vi "Analog Trigger with Interleaving Select.vi"(0 "all channels":cluster{fxp<+/-,12,1>[]}[](array[cluster])=[{[0.0, 0.0, 0.0, 0.0, 0.0, 0.0, 0.0, 0.0, 0.0, 0.0, 0.0, 0.0, 0.0, 0.0, 0.0, 0.0]}, {[0.0, 0.0, 0.0, 0.0, 0.0, 0.0, 0.0, 0.0, 0.0, 0.0, 0.0, 0.0, 0.0, 0.0, 0.0, 0.0]}], 1 "interleaving factor":u16, 5 "channel":fxp<+,2,2> format="%#_4g", 7 "trigger level":fxp<+/-,32,1>, 9 "hysteresis level":fxp<+/-,32,1>, 11 "rising edge":bool=TRUE) -> (4 "all channels delayed":cluster{fxp<+/-,12,1>[]}[](array[cluster]), 6 "triggered":bool)   [LabVIEW 2020, in "GettingStarted_5774_FPGA.lvlib"]
uses:
  GettingStarted_5774_FPGA.lvlib
  db24aacc-3aa9-45e6-b75f-233848c1dcdd.vi
  1961724d-2c00-4db4-be5f-47e2776cd38e.vi
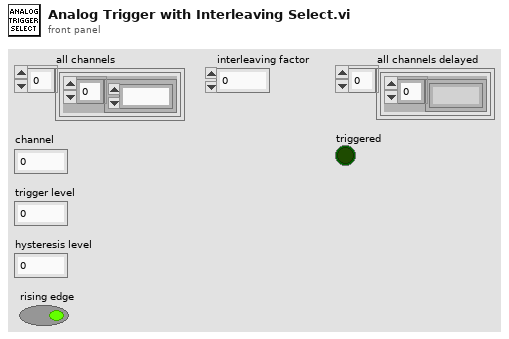
[diagram p1: front panel]
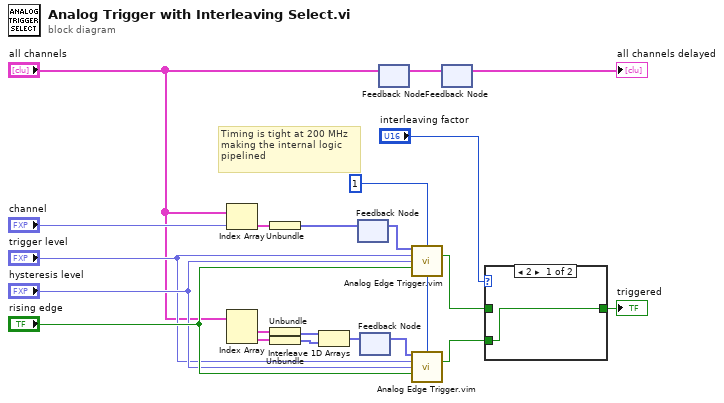
[diagram p0: block diagram]
diagram:
  w4 = u8 1 ("internal pipeline stages")
  # "Timing is tight at 200 MHz\nmaking the internal logic \npipelined"
  n1 = Index Array(array="all channels", index="channel") -> (element=w13:cluster{fxp<+/-,12,1>[]})
  n2 = Index Array(array="all channels") -> (element #1=w16:cluster{fxp<+/-,12,1>[]}, element #2=w17:cluster{fxp<+/-,12,1>[]})  [unwired: 2 in]
  n3 = Unbundle(w13) -> (w14:fxp<+/-,12,1>[])
  n4 = Unbundle(w16) -> (w18:fxp<+/-,12,1>[])
  n5 = Unbundle(w17) -> (w19:fxp<+/-,12,1>[])
  n6 = Interleave 1D Arrays(w18, w19) -> (w20:fxp<+/-,12,1>[])
  n7 = feedback #1() -> (w12:fxp<+/-,12,1>[])  [unwired: 1 in]
  n8 = feedback-in #1(w14) -> ()
  n9 = feedback #2() -> (w15:fxp<+/-,12,1>[])  [unwired: 1 in]
  n10 = feedback-in #2(w20) -> ()
  n11 = feedback-in #3("all channels") -> ()
  n12 = feedback #3() -> (w2:cluster{fxp<+/-,12,1>[]}[])  [unwired: 1 in]
  n13 = call "Analog Edge Trigger.vim"("trigger channel data"=w12, "internal pipeline stages"=w4, "requested trigger level"="trigger level", "requested hysteresis level"="hysteresis level", "rising edge"="rising edge") -> ("triggered"=w6:bool)  [unwired: 7 in, 3 out]
  n14 = call "Analog Edge Trigger.vim"("trigger channel data"=w15, "internal pipeline stages"=w4, "requested trigger level"="trigger level", "requested hysteresis level"="hysteresis level", "rising edge"="rising edge") -> ("triggered"=w7:bool)  [unwired: 7 in, 3 out]
  n15 = feedback #4() -> (→"all channels delayed":cluster{fxp<+/-,12,1>[]}[])  [unwired: 1 in]
  n16 = feedback-in #4(w2) -> ()
  n17 = case shown="2" "interleaving factor" {
    tunnel: w7 -> [w22 _]
    tunnel: [w22 w23] -> w5
    tunnel: w6 -> [_ w23]
    frame 2 {
    }
    frame 1, Default {
    }
  }
  "triggered" <- w5
